vi "Config BERT Trigger.vi"(5 "Delayed Bits (0)":i32, 7 "Bit Delay (F:OFF)":bool, 8 "error in (no error)":errorcluster {"code" format="%.0x"}, 9 "Cycle Count (1)":i32=1, 10 "BERT Trigger (3:TRIGGER KEY)":T1(ring)=enum."TRIGGER KEY", 11 "VISA Resource Name":refnum<visa-resource-name>) -> (0 "error out":errorcluster {"code" format="%.0x"}, 3 "VISA Resource Name Out":refnum<visa-resource-name>)   [LabVIEW 2012, in "Agilent ESG Series.lvlib"]
doc: "This VI is used to set the controls and parameters associated with the bit error rate measurements.\nSpecifically, those found in the Trigger submenu of the BERT option."
uses:
  <instrlib>/Agilent ESG Series/Agilent ESG Series.lvlib
panel:
  # "ON"
  # "OFF"
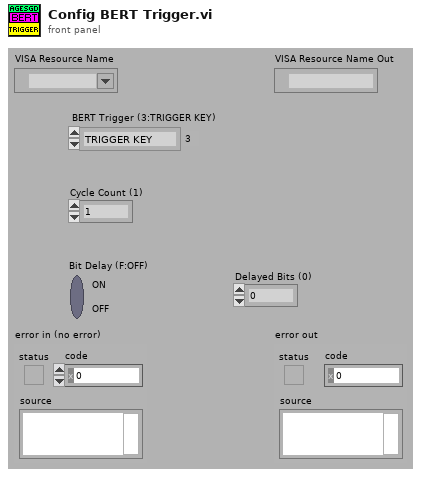
[diagram p1: front panel]
types:
  T1 = enum16{"BUS", "EXTERNAL", "IMMEDIATE", "TRIGGER KEY"}
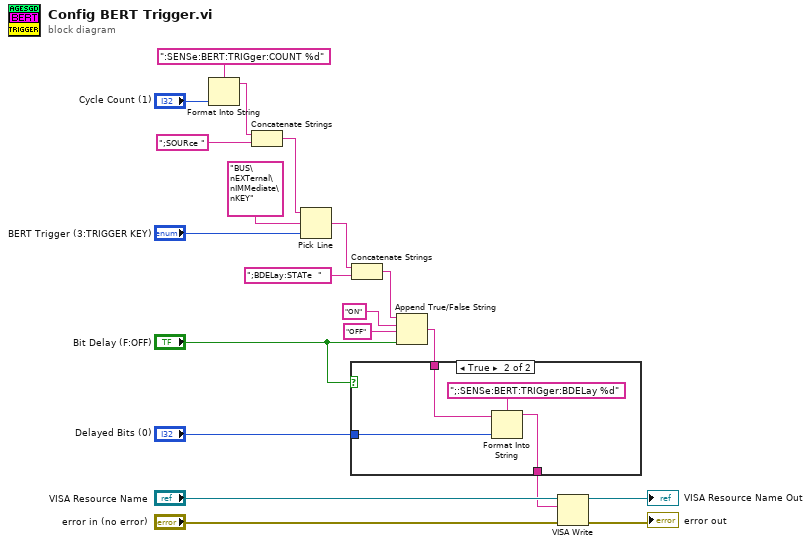
[diagram p0: block diagram]
diagram:
  n1 = Format Into String(format string=":SENSe:BERT:TRIGger:COUNT %d", "Cycle Count (1)") -> (resulting string=w13:string)  [unwired: 2 in, 1 out]
  n2 = Concatenate Strings(w13, ";SOURce ") -> (w11:string)
  n3 = Pick Line(string ("")=w11, multi-line string="BUS\nEXTernal\nIMMediate\nKEY", line index="BERT Trigger (3:TRIGGER KEY)") -> (output string=w6:string)
  n4 = Concatenate Strings(w6, ";BDELay:STATe  ") -> (w5:string)
  n5 = Append True/False String(1:"Bit Delay (F:OFF)", 2:"OFF" ("false string"), 3:"ON" ("true string"), 4:w5) -> (0:w4:string)
  n6 = case shown="True" "Bit Delay (F:OFF)" {
    tunnel: w4 -> [w21 w24]
    tunnel: "Delayed Bits (0)" -> [_ w23]
    tunnel: [w21 w22] -> w1
    frame False {
    }
    frame True {
      n7 = Format Into String(format string=";:SENSe:BERT:TRIGger:BDELay %d", initial string=w24, w23) -> (resulting string=w22:string)  [unwired: 1 in, 1 out]
    }
  }
  n8 = VISA Write(VISA resource name="VISA Resource Name", write buffer=w1, error in (no error)="error in (no error)") -> (VISA resource name out=→"VISA Resource Name Out":refnum<visa-resource-name>, error out=→"error out":errorcluster)  [unwired: 1 out]
